vi "setMatF.vi"(8 "error in (no error)":errorcluster, 9 "Matrix H":dbl[][](array[numeric]), 10 "Q Matrix":dbl[][](array[numeric]), 11 "OptCtrl in":refnum<class "OptCtrl.lvclass">) -> (0 "error out":errorcluster, 3 "OptCtrl out":refnum<class "OptCtrl.lvclass">)   [LabVIEW 2016, in "OptCtrl.lvclass"]
doc: "Set the F matrix. F = inv(A.T * C.T * C * A + rho * H)."
uses:
  OptCtrl.lvclass
  <vilib>/Analysis/baseanly.llb/Matrix Type of Inverse Matrix.ctl
  OptCtrl.lvclass/OptCtrl.ctl
  <vilib>/Analysis/Matrix/Numeric/Conversions/Array To Matrix - RA2.vi
  <vilib>/Analysis/baseanly.llb/Real Inverse Matrix.vi
  <vilib>/Analysis/Matrix/Numeric/Conversions/Matrix To Array - RM.vi
  <vilib>/Analysis/Matrix/NI_Matrix.lvlib
  <vilib>/Analysis/NI_AALBase.lvlib
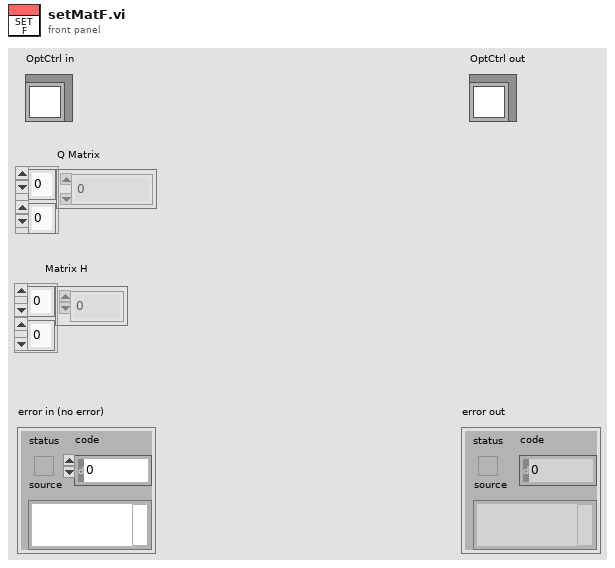
[diagram p1: front panel]
types:
  T1 = typedef "NI_AALBase.lvlib/Matrix Type of Inverse Matrix.ctl" = enum32{"General", "Positive Definite", "Lower Triangular", "Upper Triangular"}
  T2 = typedef "NI_Matrix.lvlib/RealMatrix.ctl" = dbl[][]
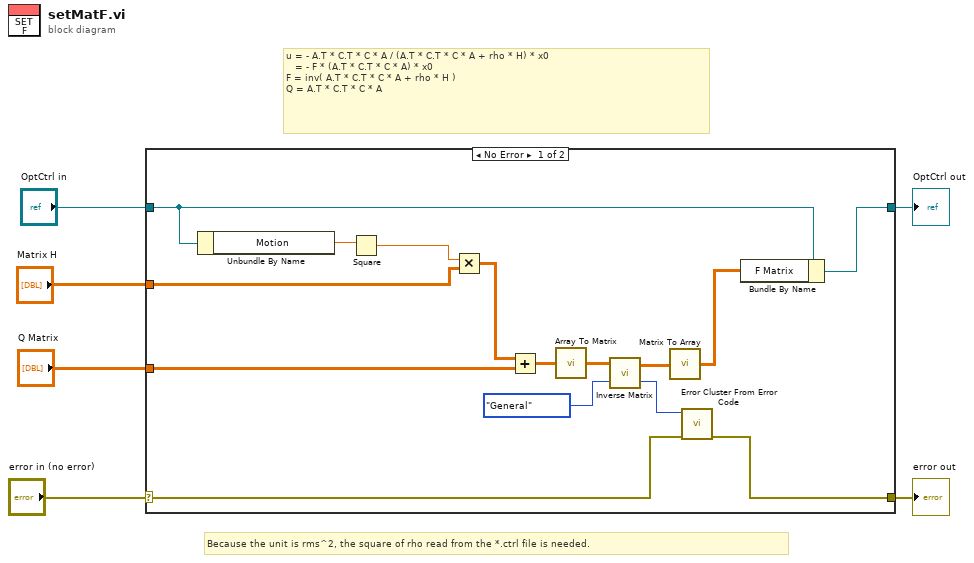
[diagram p0: block diagram]
diagram:
  # "Because the unit is rms^2, the square of rho read from the *.ctrl file is needed."
  # "u = - A.T * C.T * C * A / (A.T * C.T * C * A + rho * H) * x0\n   = - F * (A.T * C.T * C * A) * x0\nF = inv( A.T * C.T * C * A + rho * H )\nQ = A.T * C.T * C * A"
  n1 = case shown="No Error" "error in (no error)" {
    selector: "error in (no error)" -> [w7 w23]
    tunnel: [w16 w23] -> w5
    tunnel: [w13 w22] -> w3
    tunnel: "OptCtrl in" -> [w9 w22]
    tunnel: "Q Matrix" -> [w18 _]
    tunnel: "Matrix H" -> [w8 _]
    frame No Error {
      n2 = Unbundle By Name(w9) -> ("Motion"=w21:dbl)
      n3 = Square(x=w21) -> (x^2=w20:dbl)
      n4 = Multiply(x=w20, y=w8) -> (x*y=w19:dbl[][])
      n5 = Add(x=w19, y=w18) -> (x+y=w12:dbl[][])
      n6 = call-poly <vilib>:"Array To Matrix.vi"("Real 2D Array"=w12) -> ("Real Matrix"=w11:T2)
      n7 = call-poly <vilib>:"Inverse Matrix.vi"("matrix type"=Matrix_Type_of_Inverse_Matrix."General", "Input Matrix"=w11) -> ("error"=w17:i32, "Inverse Matrix"=w15:T2)
      n8 = call-poly <vilib>:"Matrix To Array.vi"("Real Matrix"=w15) -> ("Real 2D Array"=w14:dbl[][])
      n9 = call <vilib>:"Error Cluster From Error Code.vi"("error in (no error)"=w7, "error code (0)"=w17) -> ("error out"=w16:errorcluster)  [unwired: 7 in]
      n10 = Bundle By Name(cluster=w9, "F Matrix"=w14) -> (w13:refnum<class "OptCtrl.lvclass">)
    }
    frame Error {
    }
  }
  "error out" <- w5
  "OptCtrl out" <- w3
